vi "CLONE VI.vi"(7 "TRUE READ":bool, 11 "String in":string) -> (3 "String out":string)   [LabVIEW 2017]
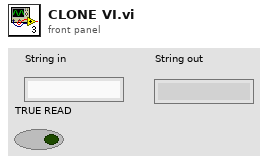
[diagram p1: front panel]
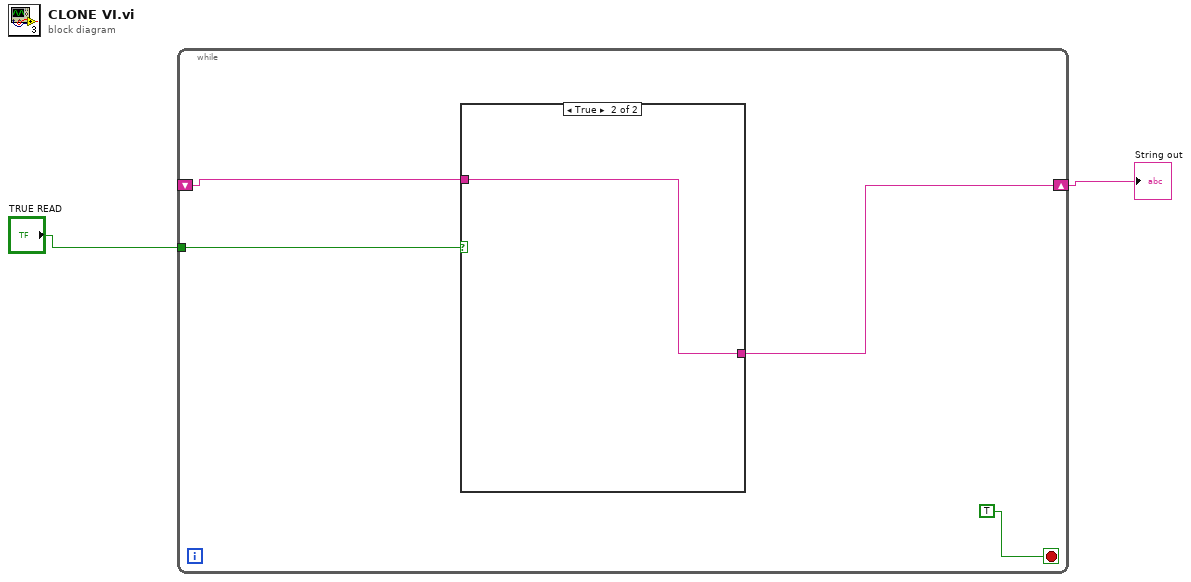
[diagram p0: block diagram]
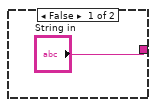
[diagram p2: hidden frame]
diagram:
  n1 = while {
    shift-right: [w6] -> w2
    shift-left: _ -> [w5]
    tunnel: "TRUE READ" -> [w4]
    stop <- TRUE stop-if-true
    n2 = case shown="True" w4 {
      tunnel: ["String in" w8] -> w6
      tunnel: w5 -> [_ w8]
      frame False {
      }
      frame True {
      }
    }
  }
  "String out" <- w2
